vi "PH_VacuumControl.Set Busy.vi"(0 "i ref in":refnum<vi>, 2 "Busy":bool, 5 "error in (no error)":errorcluster) -> (14 "i ref out":refnum<vi>, 17 "changed":bool, 19 "error out":errorcluster)   [LabVIEW 2014, in "PH_VacuumControl.lvlib"]
doc: "This VI sets the \"busy\"-flag in own attributes. If \"true\" is wanted, it checks, whether the attribute \"busy\" is already true. If so, nothing is done, and \"changed\" is false. If not, it sets the attribute and \"changed\" is true\". If \"false\" is wanted, it always sets the attribute. \n\nThis VI incluedes the \"get data to modify\" and \"set modified data\" VIs. Therefore use with care!"
uses:
  PH_VacuumControl.lvlib
  PH_Basics/PH_Common/PH_Common.lvlib
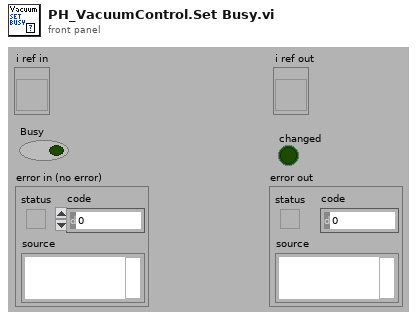
[diagram p1: front panel]
types:
  T1 = typedef "PH_VacuumControl.lvlib/PH_VacuumControl.i attribute.ctl" = cluster{"GUI Refs":cluster{"Exit":refnum<vi>, "Set Unit":refnum<vi>, "Device found":refnum<vi>, "Busy":refnum<vi>, "State":refnum<vi>, "Delete":refnum<vi>, "Channels":refnum<vi>, "Channel Name":refnum<vi>, "Trend":refnum<vi>, "Logarithmic":refnum<vi>, "Limit reached":refnum<vi>, "Channel Name 1 MT":refnum<vi>, "Channel Name 2 MT":refnum<vi>, "Trend MT":refnum<vi>, "Logarithmic MT":refnum<vi>, "Limit reached MT":refnum<vi>}, "Device found":bool, "Busy":bool, "Selected Unit":i32, "Channels [mbar]":T2, "Channel Names":cluster{"Channel 1":string, "Channel 2":string, "Channel 3":string, "Channel 4":string, "Channel 5":string, "Channel 6":string}, "Status":T3, "AGCxxx VISA Cluster":T4, "Instr Firmware Revision":string, "Service IDs Pressure":cluster{"Channel 1":i32, "Channel 2":i32, "Channel 3":i32, "Channel 4":i32, "Channel 5":i32, "Channel 6":i32}, "Service IDs Limits":cluster{"Channel 1":i32, "Channel 2":i32, "Channel 3":i32, "Channel 4":i32, "Channel 5":i32, "Channel 6":i32}, "Trend":cluster{"Start Point":timestamp, "Pressures [mbar] Channel 1":dbl[], "Pressures [mbar] Channel 2":dbl[], "Pressures [mbar] Channel 3":dbl[], "Pressures [mbar] Channel 4":dbl[], "Pressures [mbar] Channel 5":dbl[], "Pressures [mbar] Channel 6":dbl[], "Timebase [s]":i32[], "Trend Channel":u16, "Start Fit":dbl, "Trend Channel 1 MT":u16, "Trend Channel 2 MT":u16, "Start or continue Fit MT":dbl, "Continue or start Fit MT":dbl, "Datasets strored":i32, "Dataarray Size":i32}, "Running":bool}
  T2 = typedef "PH_VacuumControl.lvlib/PH_VacuumControl.Channels.ctl" = cluster{"Channel 1":dbl, "Channel 2":dbl, "Channel 3":dbl, "Channel 4":dbl, "Channel 5":dbl, "Channel 6":dbl, "Name Channel 1":string, "Name Channel 2":string, "Name Channel 3":string, "Name Channel 4":string, "Name Channel 5":string, "Name Channel 6":string, "Upper Limit":dbl, "Upper Limit 2":dbl, "Upper Limit 3":dbl, "Upper Limit 4":dbl, "Upper Limit 5":dbl, "Upper Limit 6":dbl}
  T3 = typedef "PH_StatusHandler.lvlib/PH_StatusHandler.Status.ctl" = i16
  T4 = typedef "AGCxxx - Driver.lvlib/AGCxxx VISA Control.ctl" = cluster{"VISA resource name":refnum<visa-resource-name>, "VISA Timeout Value (1000 ms)":u32, "Lock Timeout (1000 ms)":u32, "MAX Channel (6)":i32}
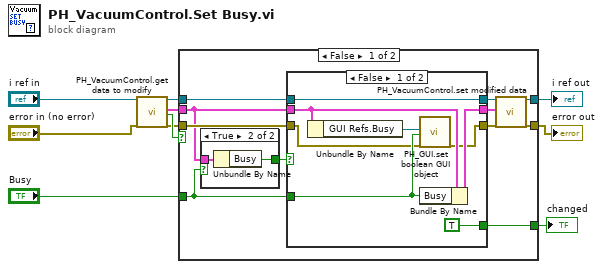
[diagram p0: block diagram]
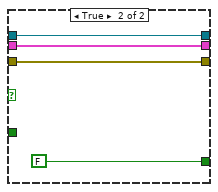
[diagram p2: hidden frame]
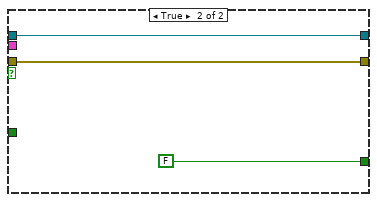
[diagram p4: hidden frame]
diagram:
  n1 = call "PH_VacuumControl.get data to modify.vi"("i ref in"="i ref in", "error in (no error)"="error in (no error)") -> ("i ref out"=w2:refnum<vi>, "i attribute"=w3:T1, "timed out"=w5:bool, "error out"=w4:errorcluster)  [unwired: 14 in]
  n2 = case shown="False" w5 {
    tunnel: w2 -> [w21 w39]
    tunnel: w3 -> [w19 _]
    tunnel: w4 -> [w20 w38]
    tunnel: [w13 w38] -> w9
    tunnel: [w15 w39] -> w10
    tunnel: "Busy" -> [w18 _]
    tunnel: [w11 FALSE] -> w1
    frame False {
      n3 = case shown="True" w18 {
        selector: w18 -> [w34 _]
        tunnel: w19 -> [_ w36]
        tunnel: [w34 w35] -> w17
        frame False {
        }
        frame True {
          n4 = Unbundle By Name(w36) -> ("Busy"=w35:bool)
        }
      }
      n5 = case shown="False" w17 {
        tunnel: w21 -> [w28 w33]
        tunnel: w20 -> [w23 w32]
        tunnel: [w22 w32] -> w14
        tunnel: [w28 w33] -> w16
        tunnel: w19 -> [w29 w31]
        tunnel: w18 -> [w24 _]
        tunnel: [w27 w31] -> w12
        tunnel: [TRUE FALSE] -> w11
        frame False {
          n6 = Unbundle By Name(w29) -> ("GUI Refs.Busy"=w25:refnum<vi>)
          n7 = call "PH_GUI.set boolean GUI object.vi"("Boolean Knob GUI Ref"=w25, "Value"=w24, "error in (no error)"=w23) -> ("error out"=w22:errorcluster)  [unwired: 16 in]
          n8 = Bundle By Name(cluster=w29, "Busy"=w24) -> (w27:T1)
        }
        frame True {
        }
      }
      n9 = call "PH_VacuumControl.set modified data.vi"("i ref in"=w16, "i attribute"=w12, "error in (no error)"=w14) -> ("i ref out"=w15:refnum<vi>, "error out"=w13:errorcluster)  [unwired: 15 in]
    }
    frame True {
    }
  }
  "i ref out" <- w10
  "error out" <- w9
  "changed" <- w1
